vi "GetControlValue.vi"(0 "vi":string, 1 "application reference (local)":refnum<vi>, 2 "vi ref":refnum<vi>, 3 "UseEnum (true)":bool=TRUE, 5 "ctrl":string, 11 "error in (no error)":errorcluster, 12 "control ref":refnum<vi>) -> (4 "String out":string, 6 "value":variant, 15 "error out":errorcluster)   [LabVIEW 2019]
uses:
  Variant/VariantArrayAccessMulti.vi
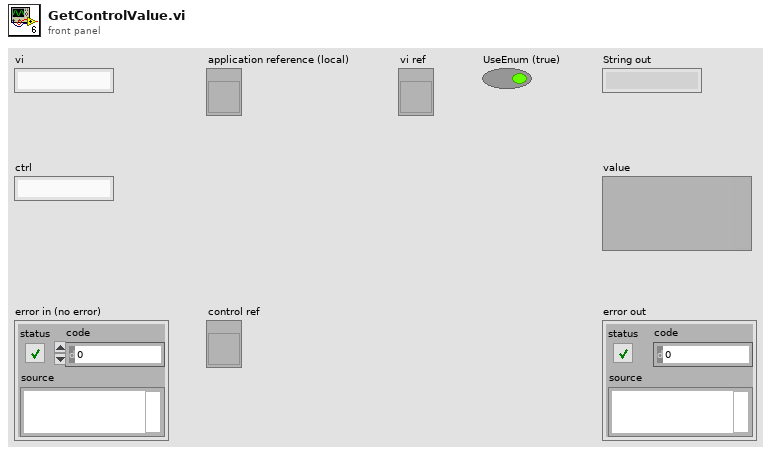
[diagram p1: front panel]
types:
  T1 = cluster{"ControlIndex":i32, "Control":refnum<vi>, "ArrayIndices":i32[]}[]
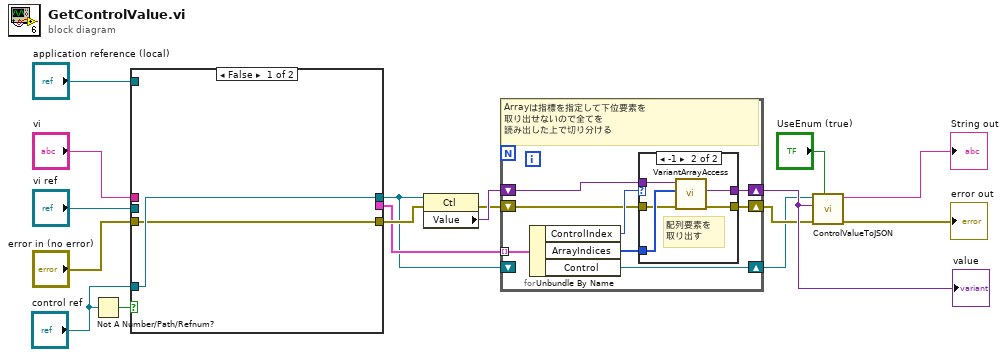
[diagram p0: block diagram]
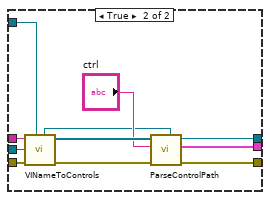
[diagram p2: hidden frame]
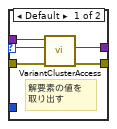
[diagram p3: hidden frame]
diagram:
  n1 = Not A Number/Path/Refnum?(number/path/refnum="control ref") -> (NaN/Path/Refnum?=w2:bool)
  n2 = case shown="False" w2 {
    tunnel: "application reference (local)" -> [_ w30]
    tunnel: "vi" -> [_ w29]
    tunnel: "error in (no error)" -> [w18 w28]
    tunnel: [w18 w23] -> w9
    tunnel: [_ w22] -> w8
    tunnel: [w19 w21] -> w5
    tunnel: "vi ref" -> [_ w20]
    tunnel: "control ref" -> [w19 _]
    frame False {
    }
    frame True {
      n3 = call "VINameToControls.vi"("application reference (local)"=w30, "error in (no error)"=w28, "vi ref"=w20, "vi"=w29) -> ("error out"=w25:errorcluster, "FlattenControls[]"=w27:refnum<vi>[], "VI out"=w24:refnum<vi>)  [unwired: 5 in]
      n4 = call "ParseControlPath.vi"("VI"=w24, "error in (no error)"=w25, "control path string"="ctrl", "Controls[]"=w27) -> ("error out"=w23:errorcluster, "subcontrol path"=w22:T1, "control"=w21:refnum<vi>)  [unwired: 4 in, 1 out]
    }
  }
  n5 = property class="Ctl"(reference=w5, error in=w9) -> (error out=w10:errorcluster, "Value"=w11:variant)  [unwired: 1 out]
  n6 = for {
    shift-right: [w37] -> w7
    shift-left: w11 -> [w34]
    tunnel: w8 -> [w38] mode=indexing
    shift-right: [w36] -> w6
    shift-left: w10 -> [w33]
    shift-right: [w31] -> w4
    shift-left: w5 -> [_]
    # "Arrayは指標を指定して下位要素を\n取り出せないので全てを\n読み出した上で切り分ける"
    n7 = Unbundle By Name(w38) -> ("ControlIndex"=w35:i32, "ArrayIndices"=w32:i32[], "Control"=w31:refnum<vi>)
    n8 = case shown="-1" w35 {
      selector: w35 -> [w39 _]
      tunnel: w34 -> [w43 w48]
      tunnel: w33 -> [w42 w46]
      tunnel: [w41 w45] -> w37
      tunnel: [w40 w44] -> w36
      tunnel: w32 -> [_ w47]
      frame Default {
        # "解要素の値を\n取り出す"
        n9 = call "VariantClusterAccess.vi"("error in (no error)"=w42, "index"=w39, "Cluster Variable"=w43) -> ("error out"=w40:errorcluster, "value"=w41:variant)  [unwired: 4 in, 3 out]
      }
      frame -1 {
        # "配列要素を\n取り出す"
        n10 = call-poly "VariantArrayAccess.vi"("error in (no error)"=w46, "Indices"=w47, "Array"=w48) -> ("error out"=w44:errorcluster, "value"=w45:variant)  [unwired: 3 in, 4 out]
      }
    }
  }
  "value" <- w7
  n11 = call "ControlValueToJSON.vi"("UseEnum"="UseEnum (true)", "error in (no error)"=w6, "Value"=w7, "Control in"=w4) -> ("error out"=→"error out":errorcluster, "String"=→"String out":string)  [unwired: 6 in]
